vi "Autonomous Block Template.vi"() -> ()   [LabVIEW 2011]
panel:
  out "Done Executing":bool
  in  "Execute":bool
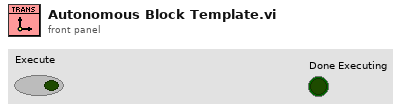
[diagram p1: front panel]
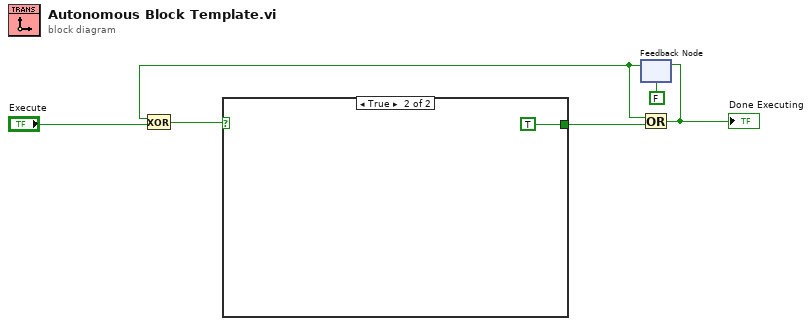
[diagram p0: block diagram]
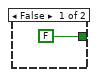
[diagram p2: hidden frame]
diagram:
  n1 = feedback #1(FALSE) -> (w2:bool)
  n2 = Exclusive Or(1:"Execute", 2:w2) -> (0:w6:bool)
  n3 = case shown="True" w6 {
    tunnel: [FALSE TRUE] -> w4
    frame False {
    }
    frame True {
    }
  }
  n4 = Or(x=w2, y=w4) -> (x .or. y?=w3:bool)
  "Done Executing" <- w3
  n5 = feedback-in #1(w3) -> ()
